vi "Read AllDisabledColumns.vi"(8 "error in (no error)":errorcluster, 11 "MenuDisableCol in":refnum<class "MenuDisableCol.lvclass">) -> (0 "error out":errorcluster, 2 "AllDisabledColumns":dbl[](array[numeric]), 3 "MenuDisableCol out":refnum<class "MenuDisableCol.lvclass">)   [LabVIEW 2013, in "MenuDisableCol.lvclass"]
uses:
  MenuDisableCol.lvclass
  MenuDisableCol.lvclass/MenuDisableCol.ctl
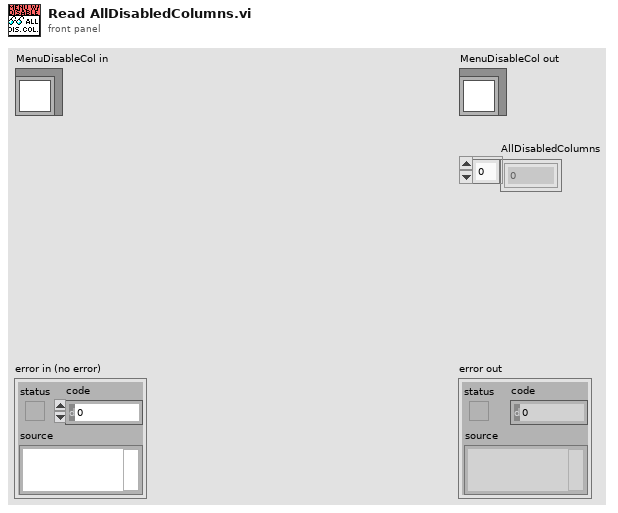
[diagram p1: front panel]
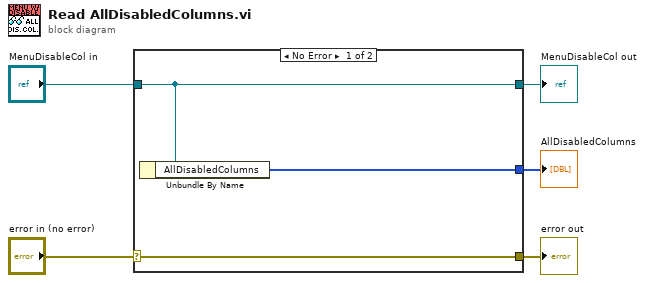
[diagram p0: block diagram]
diagram:
  n1 = case shown="No Error" "error in (no error)" {
    selector: "error in (no error)" -> [w8 w9]
    tunnel: [w8 w9] -> w4
    tunnel: [w7 w10] -> w2
    tunnel: "MenuDisableCol in" -> [w7 w10]
    tunnel: [w6 _] -> w1
    frame No Error {
      n2 = Unbundle By Name(w7) -> ("AllDisabledColumns"=w6:i32[])
    }
    frame Error {
    }
  }
  "error out" <- w4
  "MenuDisableCol out" <- w2
  "AllDisabledColumns" <- w1
